vi "Write ByRef (Unnamed SEQ).vi"(8 "error in (no error)":errorcluster, 10 "ByRef (Unnamed SEQ)":i32, 11 "MementoNumeric in":refnum<class "MementoNumeric.lvclass">) -> (0 "error out":errorcluster, 3 "MementoNumeric out":refnum<class "MementoNumeric.lvclass">)   [LabVIEW 2009, in "MementoNumeric.lvclass"]
uses:
  MementoNumeric.lvclass
  MementoNumeric.lvclass/MementoNumeric.ctl
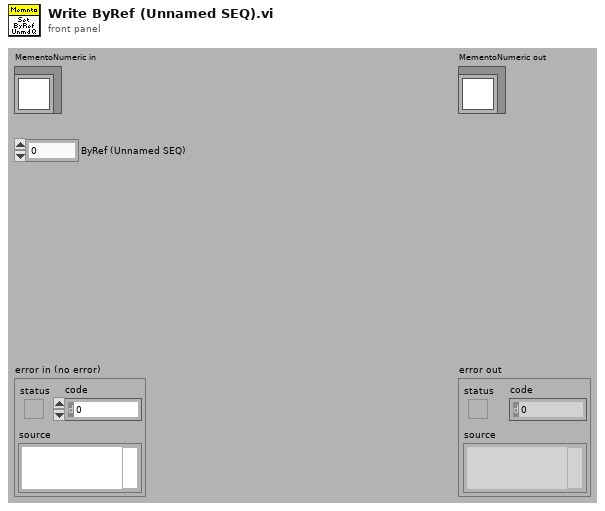
[diagram p1: front panel]
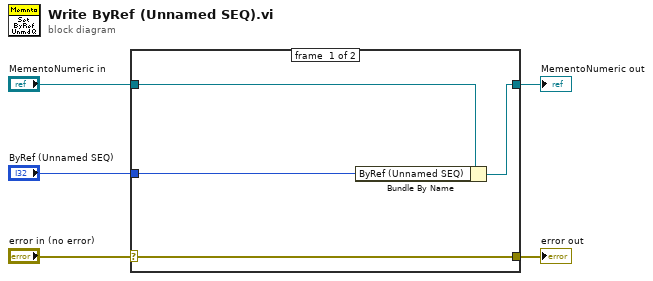
[diagram p0: block diagram]
diagram:
  n1 = case shown="No Error" "error in (no error)" {
    selector: "error in (no error)" -> [w9 w10]
    tunnel: [w9 w10] -> w4
    tunnel: [w7 w11] -> w2
    tunnel: "MementoNumeric in" -> [w8 w11]
    tunnel: "ByRef (Unnamed SEQ)" -> [w6 _]
    frame #0 {
      n2 = Bundle By Name(cluster=w8, "ByRef (Unnamed SEQ)"=w6) -> (w7:refnum<class "MementoNumeric.lvclass">)
    }
    frame #1 {
    }
  }
  "error out" <- w4
  "MementoNumeric out" <- w2
